vi "FTW-Endpoint-Receive.vi"(0 "FTW Endpoint":refnum<class "FTW-Endpoint.lvclass">, 5 "Timeout":i32 format="%dmsec", 11 "error in":errorcluster) -> (4 "FTW Endpoint out":refnum<class "FTW-Endpoint.lvclass">, 6 "Message Header":string, 8 "Message Body":string, 10 "Timed out?":bool, 15 "error out":errorcluster)   [LabVIEW 2013, in "FTW-Actor.lvlib" / "FTW-Endpoint.lvclass"]
uses:
  FTW-Endpoint.lvclass
  Request/FTW-Request.lvclass
panel:
  # "Inputs"
  # "Outputs"
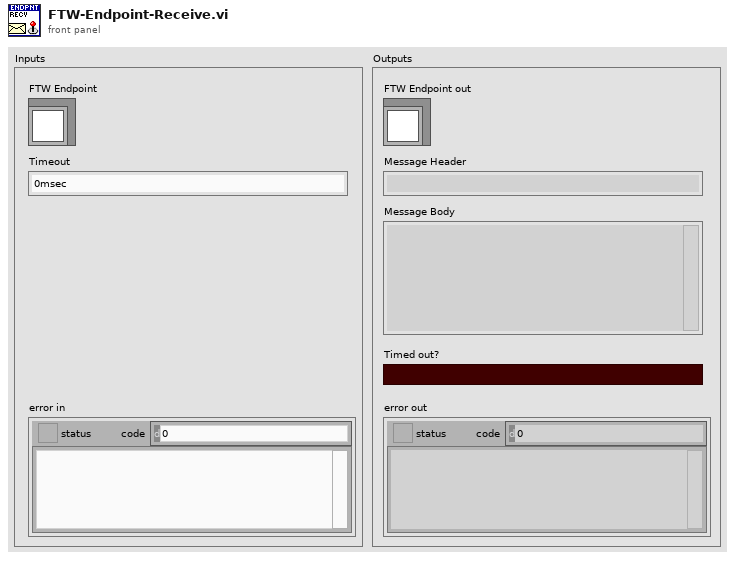
[diagram p1: front panel]
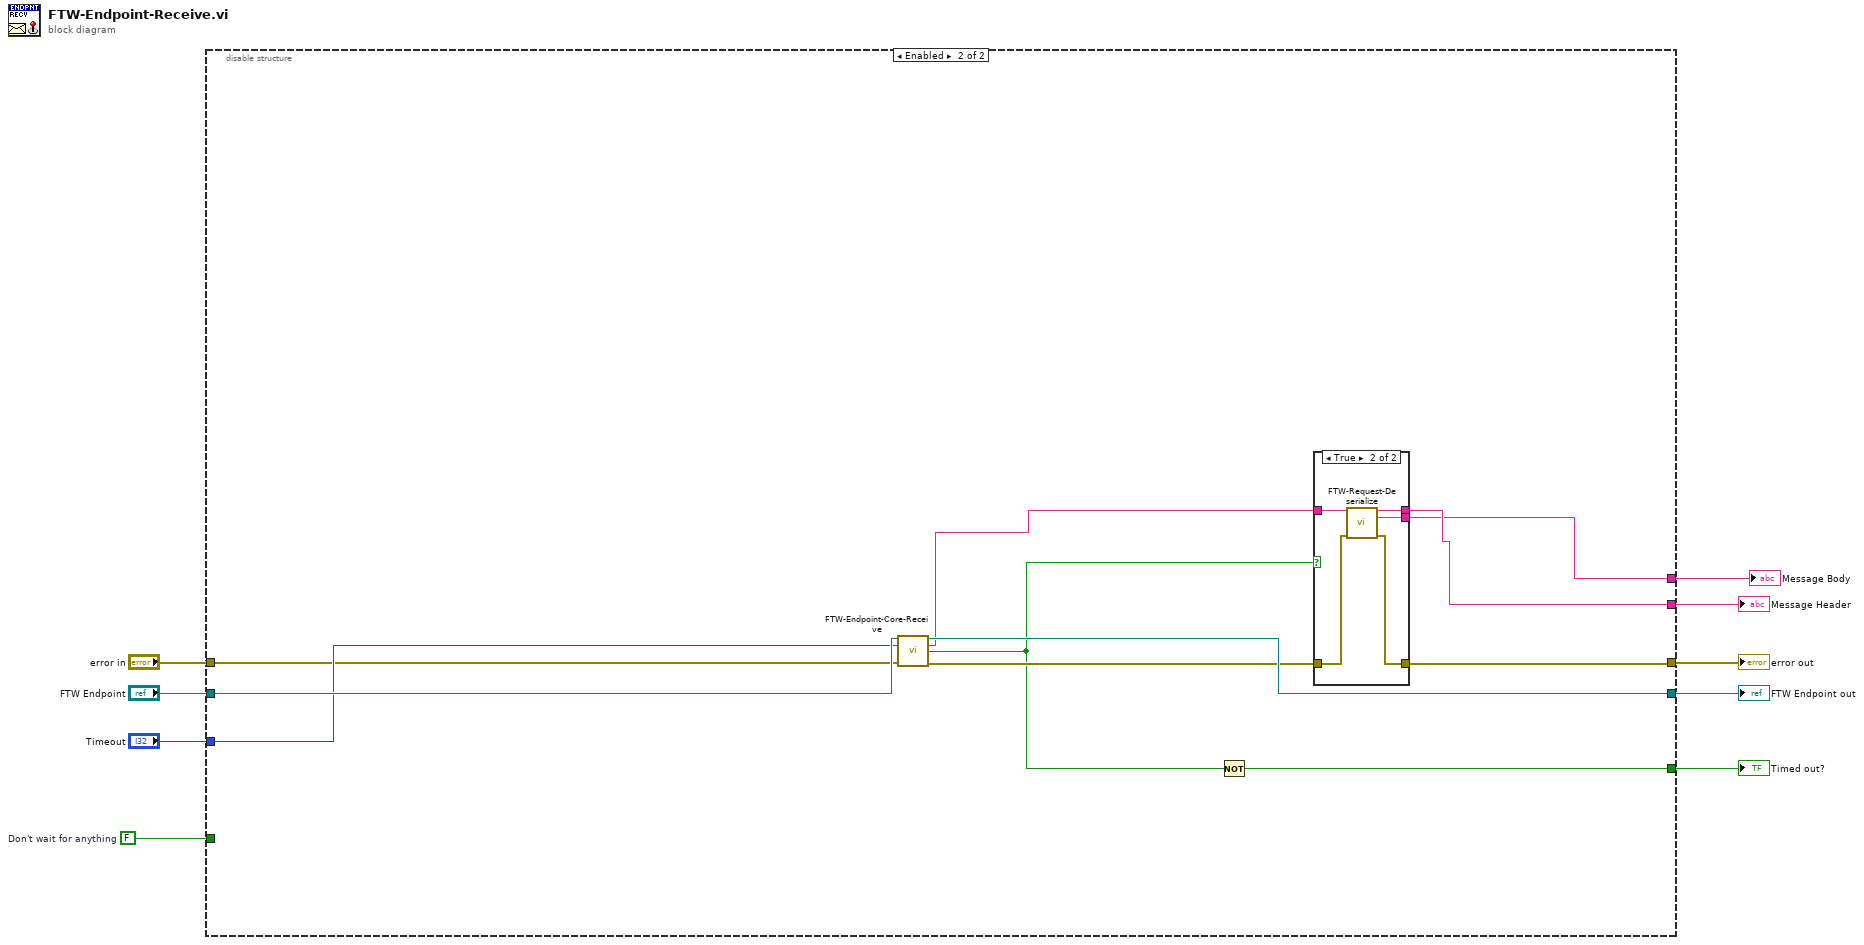
[diagram p0: block diagram]
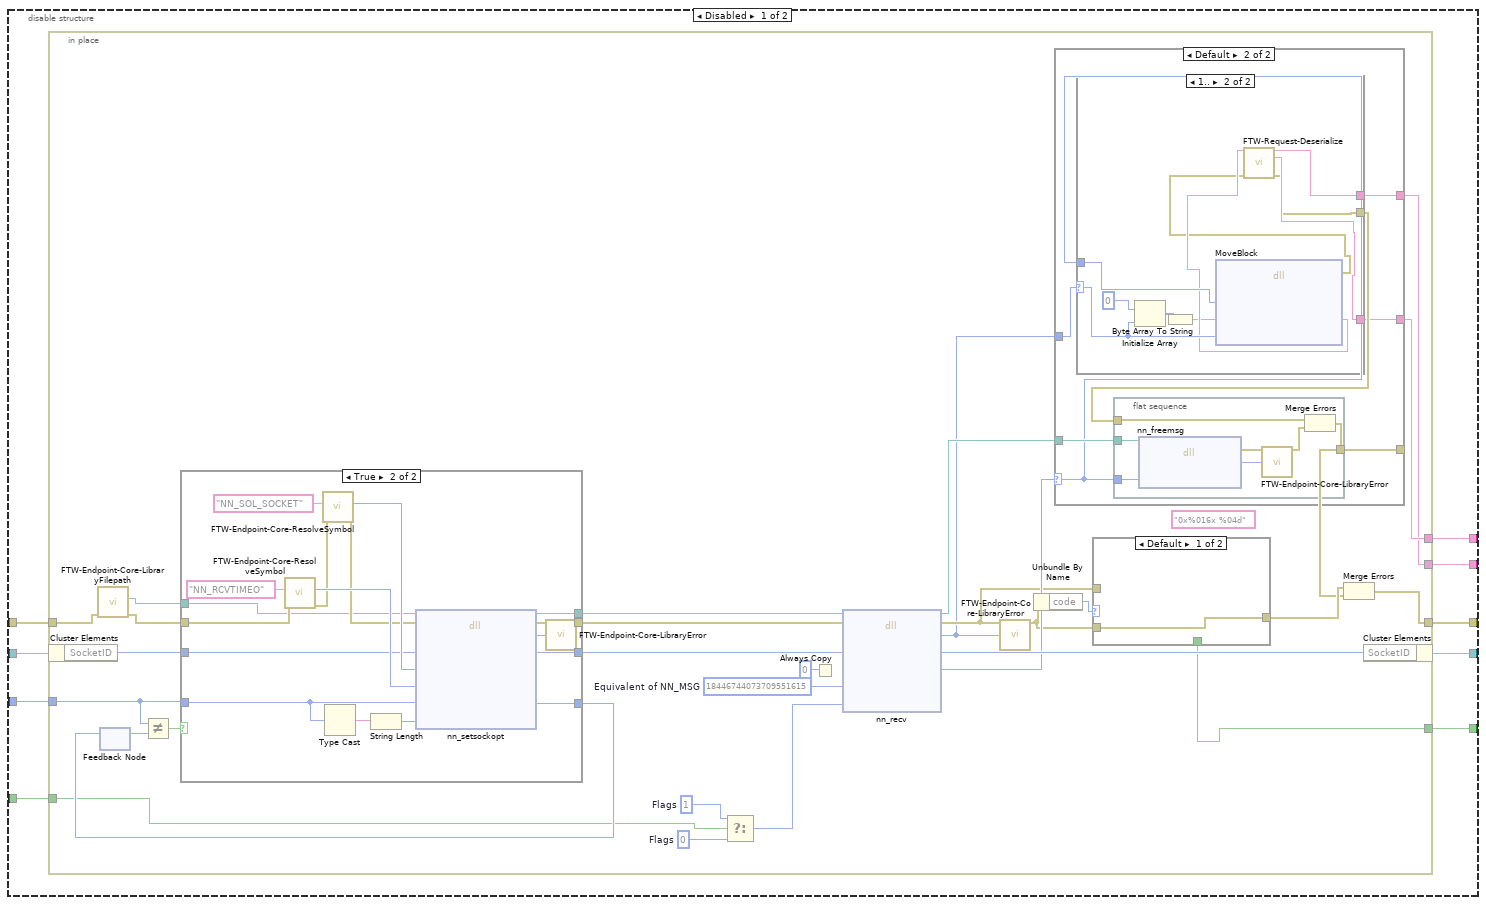
[diagram p2: hidden frame]
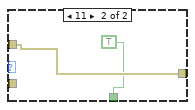
[diagram p4: hidden frame]
diagram:
  w2 = FALSE  # Don't wait for anything
  n1 = disable-structure shown="Enabled" {
    disable-tunnel: "error in" -> [w18 w106]
    disable-tunnel: [w17 w100] -> w8
    disable-tunnel: "FTW Endpoint" -> [w16 w108]
    disable-tunnel: [w15 w104] -> w6
    disable-tunnel: [w14 w102] -> w5
    disable-tunnel: [w13 w103] -> w4
    disable-tunnel: "Timeout" -> [w12 w107]
    disable-tunnel: w2 -> [w11 _]
    disable-tunnel: [w10 w105] -> w1
    frame Disabled {
      n2 = in-place {
        in-place-border: w18 -> [w29]
        in-place-border: [w36] -> w17
        in-place-border: [w25] -> w14
        in-place-border: w12 -> [w32]
        in-place-border: [w24] -> w13
        in-place-border: w11 -> [w21]
        in-place-border: [w19] -> w10
        w22 = 0  # Flags
        (unwired) "0x%016x %04d" ("format string")
        w47 = u64 18446744073709551615  # Equivalent of NN_MSG
        w23 = 1  # Flags
        n3 = in-place-cluster #1(w16) -> ("SocketID"=w45:i64)
        n4 = call "FTW-Endpoint-Core-LibraryFilepath.vi"("error in"=w29) -> ("error out"=w28:errorcluster, "Library Filepath"=w27:path)  [unwired: 8 in, 1 out]
        n5 = feedback #2() -> (w33:i32)  [unwired: 1 in]
        n6 = Not Equal?(x=w32, y=w33) -> (x != y?=w30:bool)
        n7 = case shown="True" w30 {
          tunnel: w28 -> [w52 w54]
          tunnel: w45 -> [w51 w63]
          tunnel: [w51 w62] -> w44
          tunnel: [w52 w60] -> w43
          tunnel: [w49 w59] -> w42
          tunnel: w32 -> [w50 w56]
          tunnel: [w50 w55] -> w31
          tunnel: w27 -> [w49 w53]
          frame False {
          }
          frame True {
            n8 = call "FTW-Endpoint-Core-ResolveSymbol.vi"("error in"=w54, "Symbol"="NN_RCVTIMEO") -> ("error out"=w64:errorcluster, "Symbol Value"=w67:i32)  [unwired: 8 in]
            n9 = call "FTW-Endpoint-Core-ResolveSymbol.vi"("error in"=w64, "Symbol"="NN_SOL_SOCKET") -> ("error out"=w61:errorcluster, "Symbol Value"=w65:i32)  [unwired: 8 in]
            n10 = Type Cast(x=w56) -> (*(type *) &x=w58:string)  [unwired: 1 in]
            n11 = String Length(string=w58) -> (length=w57:i32)
            n12 = dll-call lib="?" fn="nn_setsockopt"(path in=w53, error in=w61, "SocketID"=w63, "Option Level"=w65, "Option"=w67, "Option Value"=w56, "Option Value Length"=w57) -> (path out=w59:path, error out=w69:errorcluster, "Return Value"=w70:i64, "SocketID"=w62:i64, "Option Value"=w55:i32)  [unwired: 4 in]
            n13 = call "FTW-Endpoint-Core-LibraryError.vi"("error in"=w69, "Return Value"=w70) -> ("error out"=w60:errorcluster)  [unwired: 13 in]
          }
        }
        n14 = feedback-in #2(w31) -> ()
        n15 = Select(t=w23, s=w21, f=w22) -> (s? t:f=w20:i32)
        n16 = Always Copy(1:i64 0 ("buf")) -> ()  [unwired: 1 out]
        n17 = dll-call lib="?" fn="nn_recv"(path in=w42, error in=w43, "SocketID"=w44, "Message Length"=w47, "Flags"=w20) -> (path out=w46:path, error out=w34:errorcluster, "Return Value"=w26:i64, "SocketID"=w48:i64, "Message Pointer"=w40:i64)  [unwired: 4 in]
        n18 = call "FTW-Endpoint-Core-LibraryError.vi"("error in"=w34, "Return Value"=w26) -> ("error out"=w38:errorcluster)  [unwired: 13 in]
        n19 = Unbundle By Name(w38) -> ("code"=w39:i32)
        n20 = case shown="Default" w40 {
          selector: w40 -> [_ w75]
          tunnel: [_ w80] -> w35
          tunnel: w46 -> [_ w79]
          tunnel: w26 -> [_ w77]
          tunnel: [_ w76] -> w25
          tunnel: [_ w74] -> w24
          frame 0 {
          }
          frame Default {
            n21 = case shown="1.." w77 {
              selector: w77 -> [_ w88]
              tunnel: [_ w83] -> w78
              tunnel: [_ w87] -> w76
              tunnel: w75 -> [_ w90]
              tunnel: [_ w86] -> w74
              frame ..0 {
              }
              frame 1.. {
                n22 = Initialize Array(u8 0, w88) -> (w82:u8[])
                n23 = Byte Array To String(unsigned byte array=w82) -> (string=w81:string)
                n24 = dll-call lib="LabVIEW" fn="MoveBlock"("Source Pointer"=w90, "Pointer to Destination"=w81, "String Length"=w88) -> (error out=w84:errorcluster, "Pointer to Destination"=w85:string)  [unwired: 6 in, 1 out]
                n25 = call "FTW-Request-Deserialize.vi"("Message"=w85, "error in"=w84) -> ("Message Header"=w86:string, "Message Body"=w87:string, "error out"=w83:errorcluster)  [unwired: 11 in]
              }
            }
            n26 = flat-sequence {
              tunnel: [w91] -> w80
              tunnel: w79 -> [w95]
              tunnel: w75 -> [w94]
              tunnel: w78 -> [w92]
              frame #0 {
                n27 = dll-call lib="?" fn="nn_freemsg"(path in=w95, "Message Pointer"=w94) -> (error out=w97:errorcluster, "Return Value"=w96:i64)  [unwired: 3 in, 1 out]
                n28 = call "FTW-Endpoint-Core-LibraryError.vi"("error in"=w97, "Return Value"=w96) -> ("error out"=w93:errorcluster)  [unwired: 13 in]
                n29 = Merge Errors(w92, w93) -> (w91:errorcluster)
              }
            }
          }
        }
        n30 = case shown="Default" w39 {
          tunnel: [w71 w73] -> w37
          tunnel: w38 -> [w71 _]
          tunnel: w34 -> [_ w73]
          tunnel: [_ TRUE] -> w19
          frame Default {
          }
          frame 11 {
          }
        }
        n31 = Merge Errors(w37, w35) -> (w36:errorcluster)
        n32 = in-place-cluster #1("SocketID"=w48) -> (w15:refnum<class "FTW-Endpoint.lvclass">)
      }
    }
    frame Enabled {
      n33 = call "FTW-Endpoint-Core-Receive.vi"("FTW Endpoint"=w108, "Timeout"=w107, "error in"=w106) -> ("FTW Endpoint out"=w104:refnum<class "FTW-Endpoint.lvclass">, "Message"=w99:string, "Message Received?"=w98:bool, "error out"=w101:errorcluster)  [unwired: 7 in, 2 out]
      n34 = Not(x=w98) -> (.not. x?=w105:bool)
      n35 = case shown="True" w98 {
        tunnel: [_ w114] -> w103
        tunnel: [_ w113] -> w102
        tunnel: w101 -> [w109 w112]
        tunnel: [w109 w111] -> w100
        tunnel: w99 -> [_ w110]
        frame False {
        }
        frame True {
          n36 = call "FTW-Request-Deserialize.vi"("Message"=w110, "error in"=w112) -> ("Message Header"=w114:string, "Message Body"=w113:string, "error out"=w111:errorcluster)  [unwired: 11 in]
        }
      }
    }
  }
  "error out" <- w8
  "FTW Endpoint out" <- w6
  "Timed out?" <- w1
  "Message Header" <- w4
  "Message Body" <- w5
